vi "ConfigFile Name.vi"() -> (1 "ConfigFile Name":string)   [LabVIEW 2009]
uses:
  <vilib>/regexp/Match Regular Expression.xnode
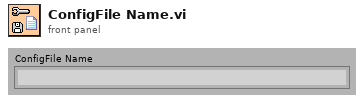
[diagram p1: front panel]
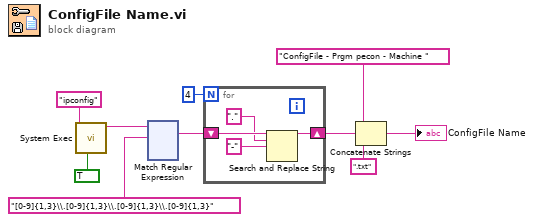
[diagram p0: block diagram]
diagram:
  n1 = call <vilib>:"System Exec.vi"("run minimized? (F)"=TRUE, "command line"="ipconfig") -> ("standard output"=w2:string)  [unwired: 6 in, 3 out]
  n2 = xnode "Match Regular Expression"("input string"=w2, "regular expression"="[0-9]{1,3}\\.[0-9]{1,3}\\.[0-9]{1,3}\\.[0-9]{1,3}") -> ("whole match"=w5:string)  [unwired: 4 in, 4 out]
  n3 = for {
    N: 4 -> [_]
    shift-right: [w13] -> w8
    shift-left: w5 -> [w14]
    n4 = Search and Replace String(input string=w14, search string=".", replace string="-" ("replace string (\"\")")) -> (result string=w13:string)  [unwired: 5 in, 3 out]
  }
  n5 = Concatenate Strings("ConfigFile - Prgm pecon - Machine " ("string"), w8, ".txt" ("string")) -> (→"ConfigFile Name":string)
